vi "onInterruptProcessTriggers.vi"(8 "error in (no error)":errorcluster, 10 "model in":refnum<class "IModel.lvclass">, 11 "ImagingState in":refnum<class "ImagingState.lvclass">) -> (0 "error out":errorcluster, 2 "model out":refnum<class "IModel.lvclass">, 3 "ImagingState out":refnum<class "ImagingState.lvclass">)   [LabVIEW 2016, in "States.lvlib" / "ImagingState.lvclass"]
uses:
  ImagingState.lvclass
  IModel/IModel.lvclass
  ts_sallv_sedspectrometer/DataTypes/logevent_DetailedState.ctl
  ts_sallv_sedspectrometer/SALLV_sedSpectrometer.lvlib
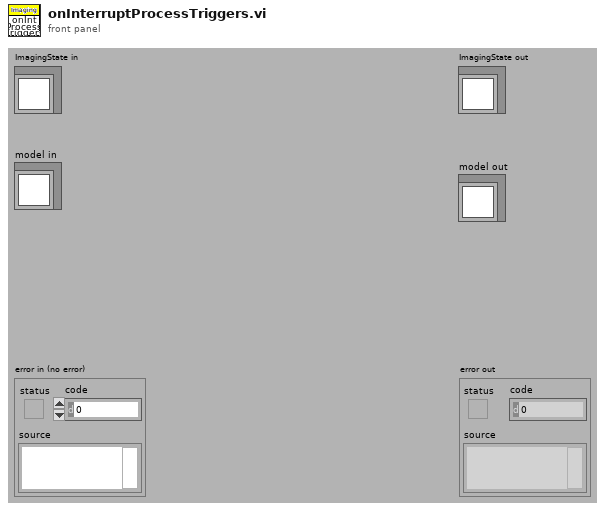
[diagram p1: front panel]
types:
  T1 = typedef "SALLV_sedSpectrometer.lvlib/logevent_DetailedState.ctl" = cluster{"detailedState":enum32{"", "DisabledState", "FaultState", "OfflineState", "StandbyState", "ImagingState", "NotImagingState"}, "priority":i32}
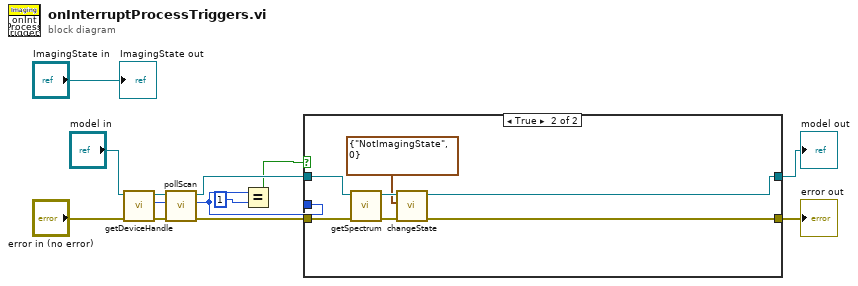
[diagram p0: block diagram]
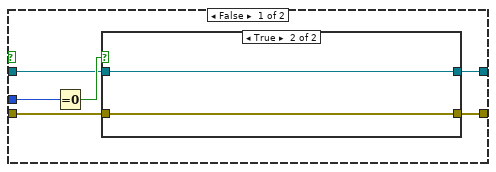
[diagram p2: hidden frame]
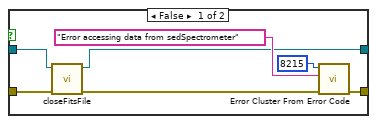
[diagram p3: hidden frame]
diagram:
  n1 = call-dynamic "getDeviceHandle.vi"("error in (no error)"="error in (no error)", "IModel in"="model in") -> ("error out"=w10:errorcluster, "Device"=w9:i32, "IModel out"=w13:refnum<class "IModel.lvclass">)  [unwired: 7 in]
  n2 = call-dynamic "pollScan.vi"("error in (no error)"=w10, "Device"=w9, "IModel in"=w13) -> ("error out"=w11:errorcluster, "Output Value"=w3:i32, "IModel out"=w12:refnum<class "IModel.lvclass">)  [unwired: 6 in]
  n3 = Equal?(x=w3, y=1) -> (x = y?=w1:bool)
  n4 = case shown="True" w1 {
    tunnel: w12 -> [w15 w35]
    tunnel: w11 -> [w17 w34]
    tunnel: [w14 w29] -> w5
    tunnel: [w16 w31] -> w4
    tunnel: w3 -> [w19 _]
    frame False {
      n5 = Equal To 0?(x=w19) -> (x = 0?=w18:bool)
      n6 = case shown="True" w18 {
        tunnel: w17 -> [w20 w28]
        tunnel: [w24 w28] -> w16
        tunnel: w15 -> [w23 w27]
        tunnel: [w22 w27] -> w14
        frame False {
          n7 = call-dynamic "closeFitsFile.vi"("error in (no error)"=w20, "IModel in"=w23) -> ("error out"=w21:errorcluster, "IModel out"=w22:refnum<class "IModel.lvclass">)  [unwired: 8 in]
          n8 = call <vilib>:"Error Cluster From Error Code.vi"("error in (no error)"=w21, "error message (\"\")"="Error accessing data from sedSpectrometer" ("error message (\"\")"), "error code (0)"=8215) -> ("error out"=w24:errorcluster)  [unwired: 6 in]
        }
        frame True {
        }
      }
    }
    frame True {
      n9 = call-dynamic "getSpectrum.vi"("error in (no error)"=w34, "IModel in"=w35) -> ("error out"=w32:errorcluster, "IModel out"=w33:refnum<class "IModel.lvclass">)  [unwired: 8 in]
      n10 = call-dynamic "changeState.vi"("error in (no error)"=w32, "DetailedState"=T1 {"detailedState"=enum."NotImagingState", "priority"=0}, "IModel in"=w33) -> ("error out"=w31:errorcluster, "IModel out"=w29:refnum<class "IModel.lvclass">)  [unwired: 7 in]
    }
  }
  "error out" <- w4
  "model out" <- w5
  "ImagingState out" <- "ImagingState in"
